vi "Remove Address.vi"(8 "error in (no error)":errorcluster, 9 "Paras In":variant, 10 "ID In":variant, 11 "Simple Map Queue Group Messenger in":refnum<class "Simple Map Queue Group Messenger.lvclass">) -> (0 "error out":errorcluster, 3 "Simple Map Queue Group Messenger out":refnum<class "Simple Map Queue Group Messenger.lvclass">)   [LabVIEW 2024, in "Simple Map Queue Group Messenger.lvclass"]
uses:
  Simple Map Queue Group Messenger.lvclass
  Simple Map Queue Group Messenger.lvclass/Simple Map Queue Group Messenger.ctl
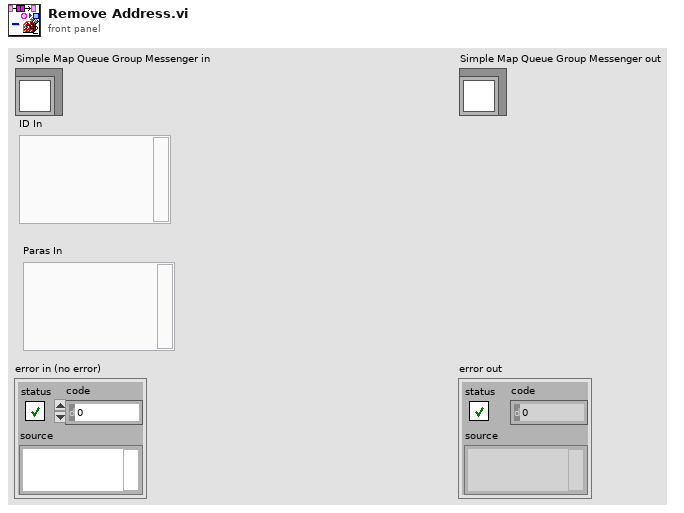
[diagram p1: front panel]
types:
  T1 = typedef "Queue Group Map.ctl" = map{i64, T2[]}
  T2 = typedef "Message Queue.ctl" = refnum<queue>
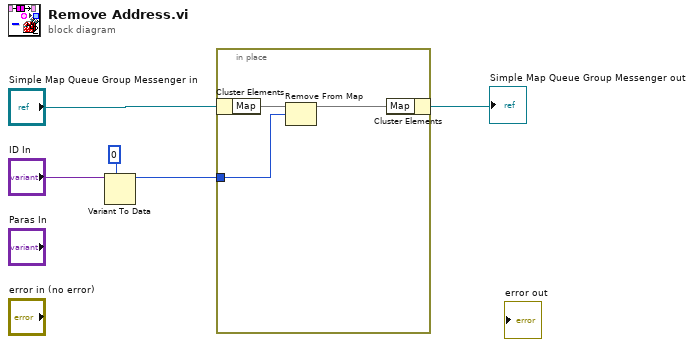
[diagram p0: block diagram]
diagram:
  n1 = Variant To Data(type=i64 0, Variant="ID In") -> (data=w1:i64)  [unwired: 1 in, 1 out]
  n2 = in-place {
    in-place-border: w1 -> [w6]
    n3 = in-place-cluster #1("Simple Map Queue Group Messenger in") -> ("Map"=w7:T1)
    n4 = Remove From Map(10:w6, 11:w7) -> (3:w8:T1)  [unwired: 2 out]
    n5 = in-place-cluster #1("Map"=w8) -> (→"Simple Map Queue Group Messenger out":refnum<class "Simple Map Queue Group Messenger.lvclass">)
  }
